vi "ZMQ Req Test.vi"() -> ()   [LabVIEW 2019, in "RemoteControl.ZMQ.lvclass"]
uses:
  RemoteControl.ZMQ.lvclass
panel:
  out "Command Sent":string
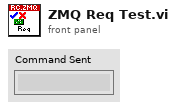
[diagram p1: front panel]
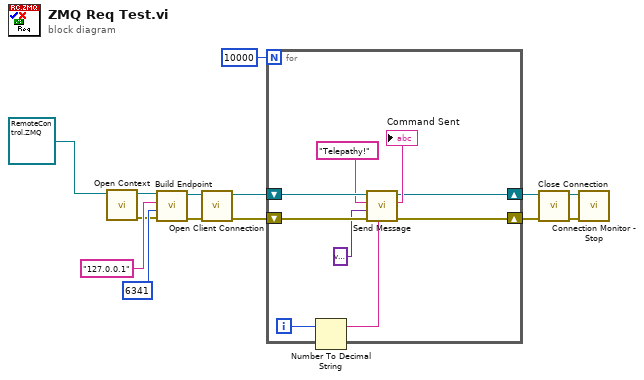
[diagram p0: block diagram]
diagram:
  n1 = call-dynamic "Open Context.vi"("RemoteControl.ZMQ in"=refnum<class "RemoteControl.ZMQ.lvclass"> refnum ("RemoteControl.ZMQ.lvclass")) -> ("error out"=w5:errorcluster, "RemoteControl.ZMQ out"=w14:refnum<class "RemoteControl.ZMQ.lvclass">)  [unwired: 9 in]
  n2 = call "Build Endpoint.vi"("error in (no error)"=w5, "Port"=u16 6341, "Address"="127.0.0.1", "RemoteControl.ZMQ in"=w14) -> ("error out"=w10:errorcluster, "RemoteControl.ZMQ out"=w11:refnum<class "RemoteControl.ZMQ.lvclass">)  [unwired: 6 in]
  n3 = call-dynamic "Open Client Connection.vi"("error in (no error)"=w10, "RemoteControl.ZMQ in"=w11) -> ("error out"=w8:errorcluster, "RemoteControl.ZMQ out"=w9:refnum<class "RemoteControl.ZMQ.lvclass">)  [unwired: 8 in]
  n4 = for {
    N: 10000 -> [_]
    shift-right: [w18] -> w4
    shift-left: w9 -> [w23]
    shift-right: [w17] -> w3
    shift-left: w8 -> [w22]
    i -> [w16]
    n5 = Number To Decimal String(number=w16) -> (decimal integer string=w15:string)  [unwired: 1 in]
    n6 = call-dynamic "Send Message.vi"("ID"=w15, "error in (no error)"=w22, "Data"=variant, "Command"="Telepathy!", "RemoteControl.ZMQ in"=w23) -> ("error out"=w17:errorcluster, "ACK"=→"Command Sent":string, "RemoteControl.ZMQ out"=w18:refnum<class "RemoteControl.ZMQ.lvclass">)  [unwired: 4 in]
  }
  n7 = call-dynamic "Close Connection.vi"("error in (no error)"=w3, "RemoteControl.ZMQ in"=w4) -> ("error out"=w6:errorcluster, "RemoteControl.ZMQ out"=w7:refnum<class "RemoteControl.ZMQ.lvclass">)  [unwired: 8 in]
  n8 = call-dynamic "Connection Monitor - Stop.vi"("error in (no error)"=w6, "RemoteControl.ZMQ in"=w7) -> ()  [unwired: 8 in, 2 out]
